vi "Initialize Notifiers.vi"(8 "error in":errorcluster) -> (0 "error out":errorcluster)   [LabVIEW 2019]
doc: "Initialize all notifiers\n\n-----\nJuan Navarro\nLab it Studio"
uses:
  Sequencer/Sequencer Handshake.lvlib
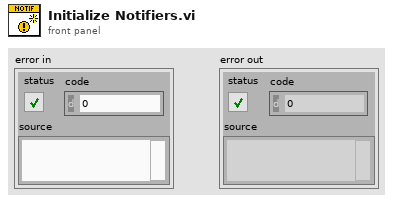
[diagram p1: front panel]
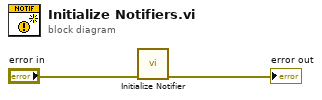
[diagram p0: block diagram]
diagram:
  n1 = call "Initialize Notifier.vi"("error in"="error in") -> ("error out"=→"error out":errorcluster)  [unwired: 10 in]
